vi "write_scan_settings_to_data_file.vi"(10 "Scan settings":T1={"Start voltage (V)"=0.01, "End voltage (V)"=200.0, "Number of steps"=44, "Settling delay (ms)"=1.0, "Dual sweep"=1, "Stabilisation time (s)"=0.0, "Stabilisation mode"=0, "Stabilisation value (V or A) "=0.0, "No. of repeat scans"=2.0, "Repeat scans"=0, "Logarithmic sweep"=1, "Electrode configuration"=0, "Sweep mode"=0, "Auto settling delay"=0, "Pulse off time (ms)"=0.0, "Integration time (ms)"=1.0, "Current range"=0, "Enable display"=0, "Enable concurrent measurements"=1, "Concurrent measurements"=1} {"Concurrent measurements" items=["Volts", "Current", "Resistance", "Volt, Current", "Volts, Resistance", "Current, Resistance", "All"]; "Enable concurrent measurements" items=["False", "True"]; "Enable display" items=["False", "True"]; "Current range" items=["Auto", "1 uA", "10 uA", "100 uA", "1 mA", "10 mA", "100 mA", "1 A"]; "Integration time (ms)" min=0.2 max=200.0; "Pulse off time (ms)" min=0.0; "Auto settling delay" items=["False", "True"]; "Sweep mode" items=["Staircase", "Pulsed"]; "Electrode configuration" items=["2-wire", "4-wire"]; "Logarithmic sweep" items=["False", "True"]; "Repeat scans" items=["False", "True"]; "No. of repeat scans" min=1.0 step=1.0; "Stabilisation mode" items=["V", "I"]; "Dual sweep" items=["False", "True"]; "Settling delay (ms)" min=0.2 max=999999.9}, 11 "file path in":path) -> (3 "file path out":path)   [LabVIEW 2016]
uses:
  TypeDefs/settings.ctl
  <vilib>/Utility/file.llb/Write Delimited Spreadsheet (string).vi
panel:
  out "Electrode configuration":u16(ring) items=["2-wire", "4-wire"]
  out "Current range":u16(ring) items=["Auto", "1 uA", "10 uA", "100 uA", "1 mA", "10 mA", "100 mA", "1 A"]
  out "Sweep mode":u16(ring) items=["Staircase", "Pulsed"]
  out "Enable concurrent measurements":u16(ring)=1 items=["False", "True"]
  out "Concurrent measurements":u16(ring)=1 items=["Volts", "Current", "Resistance", "Volt, Current", "Volts, Resistance", "Current, Resistance", "All"]
  out "scan settings":string[][](array[string])
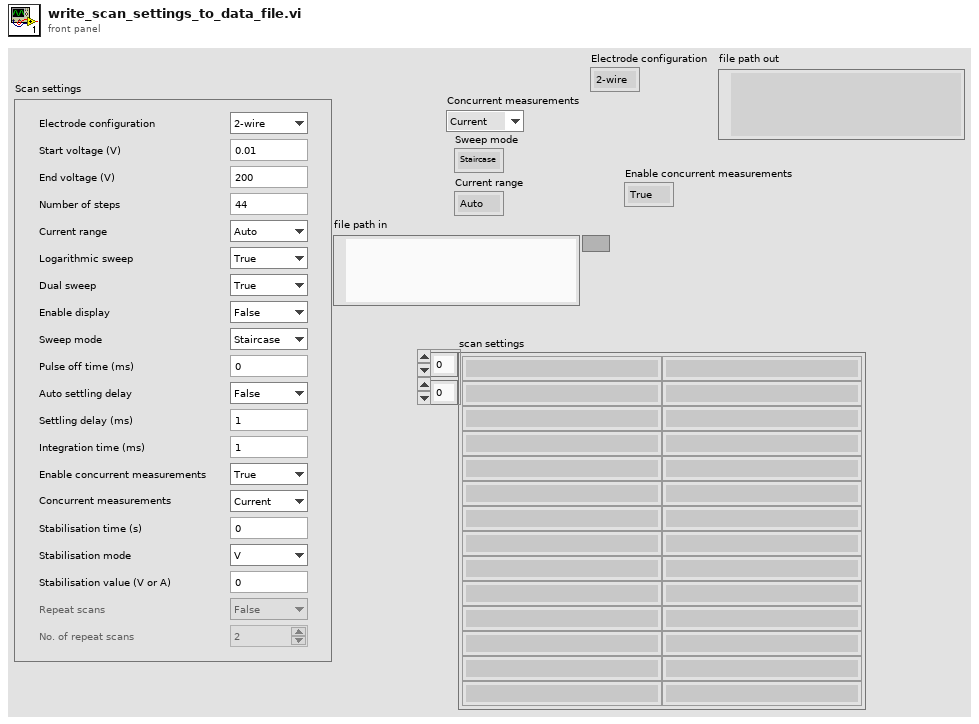
[diagram p1: front panel]
types:
  T1 = typedef "settings.ctl" = cluster{"Start voltage (V)":dbl, "End voltage (V)":dbl, "Number of steps":u32, "Settling delay (ms)":dbl, "Dual sweep":u16, "Stabilisation time (s)":dbl, "Stabilisation mode":u16, "Stabilisation value (V or A) ":dbl, "No. of repeat scans":dbl, "Repeat scans":u16, "Logarithmic sweep":u16, "Electrode configuration":u16, "Sweep mode":u16, "Auto settling delay":u16, "Pulse off time (ms)":dbl, "Integration time (ms)":dbl, "Current range":u16, "Enable display":u16, "Enable concurrent measurements":u16, "Concurrent measurements":u16}
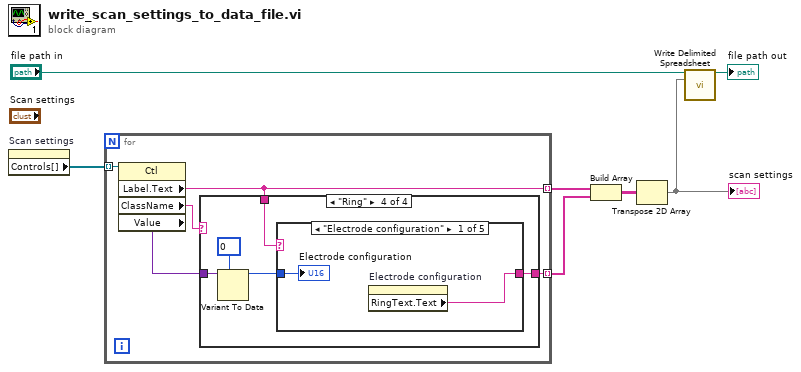
[diagram p0: block diagram]
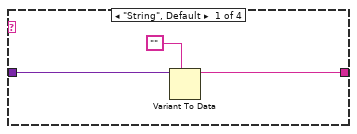
[diagram p2: hidden frame]
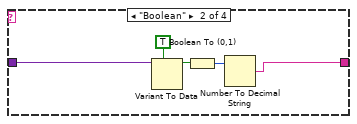
[diagram p3: hidden frame]
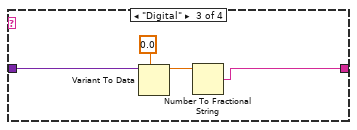
[diagram p4: hidden frame]
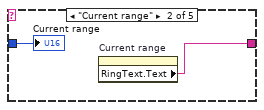
[diagram p5: hidden frame]
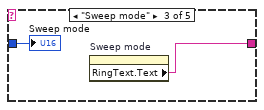
[diagram p6: hidden frame]
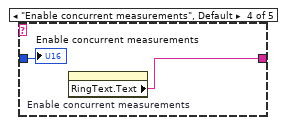
[diagram p7: hidden frame]
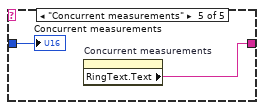
[diagram p8: hidden frame]
diagram:
  n1 = property on="Scan settings" class="Clust (strict)"() -> ("Controls[]"=w6:refnum<vi>[])  [unwired: 2 in, 2 out]
  n2 = for {
    tunnel: w6 -> [w12] mode=indexing
    tunnel: [w8] -> w7 mode=indexing
    tunnel: [w9] -> w4 mode=indexing
    n3 = property class="Ctl"(reference=w12) -> ("Label.Text"=w8:string, "ClassName"=w11:string, "Value"=w10:variant)  [unwired: 1 in, 2 out]
    n4 = case shown="\"Ring\"" w11 {
      tunnel: [w14 w17 w22 w26] -> w9
      tunnel: w10 -> [w13 w16 w21 w29]
      tunnel: w8 -> [_ _ _ w27]
      frame "String", Default {
        n5 = Variant To Data(type="", Variant=w13) -> (data=w14:string)  [unwired: 1 in, 1 out]
      }
      frame "Boolean" {
        n6 = Variant To Data(type=TRUE, Variant=w16) -> (data=w19:bool)  [unwired: 1 in, 1 out]
        n7 = Boolean To (0,1)(Boolean=w19) -> (0, 1=w18:i16)
        n8 = Number To Decimal String(number=w18) -> (decimal integer string=w17:string)  [unwired: 1 in]
      }
      frame "Digital" {
        n9 = Variant To Data(type=0.0, Variant=w21) -> (data=w23:dbl)  [unwired: 1 in, 1 out]
        n10 = Number To Fractional String(number=w23) -> (F-format string=w22:string)  [unwired: 3 in]
      }
      frame "Ring" {
        w28 = u16 0 items=[""]
        n11 = Variant To Data(type=w28, Variant=w29) -> (data=w25:u16)  [unwired: 1 in, 1 out]
        n12 = case shown="\"Electrode configuration\"" w27 {
          tunnel: [w30 w32 w34 w37 w39] -> w26
          tunnel: w25 -> [w31 w33 w35 w36 w38]
          frame "Electrode configuration" {
            n13 = property on="Electrode configuration" class="Ring (strict)"() -> ("RingText.Text"=w30:string)  [unwired: 2 in, 2 out]
            "Electrode configuration" <- w31
          }
          frame "Current range" {
            n14 = property on="Current range" class="Ring (strict)"() -> ("RingText.Text"=w32:string)  [unwired: 2 in, 2 out]
            "Current range" <- w33
          }
          frame "Sweep mode" {
            n15 = property on="Sweep mode" class="Ring (strict)"() -> ("RingText.Text"=w34:string)  [unwired: 2 in, 2 out]
            "Sweep mode" <- w35
          }
          frame "Enable concurrent measurements", Default {
            n16 = property on="Enable concurrent measurements" class="Ring (strict)"() -> ("RingText.Text"=w37:string)  [unwired: 2 in, 2 out]
            "Enable concurrent measurements" <- w36
          }
          frame "Concurrent measurements" {
            n17 = property on="Concurrent measurements" class="Ring (strict)"() -> ("RingText.Text"=w39:string)  [unwired: 2 in, 2 out]
            "Concurrent measurements" <- w38
          }
        }
      }
    }
  }
  n18 = Build Array(w7, w4) -> (w5:string[][])
  n19 = Transpose 2D Array(2D array=w5) -> (transposed array=w3:string[][])
  "scan settings" <- w3
  n20 = call-poly <vilib>:"Write Delimited Spreadsheet.vi"("file path (dialog if empty)"="file path in", "2D data"=w3) -> ("new file path (Not A Path if cancelled)"=→"file path out":path)  [unwired: 12 in, 1 out]
